vi "Check_with_Jump.vi"(4 "Model       Roll      Pitch       Yaw (deg)":dbl[](array[numeric]) format="%#.2f", 5 "Simulate/Run":T1=enum."Run VI", 6 "Exclude Array":T2[](array[typedef])=[{"Sizes"=[{"Max"=1000.0, "Min"=-1000.0}, {"Max"=1000.0, "Min"=-1000.0}, {"Max"=20.0, "Min"=0.0}], "Name"="Roughness Elements", "Exclude Type"=enum."Allow only vertical moves"}, {"Sizes"=[{"Max"=50.0, "Min"=-50.0}, {"Max"=50.0, "Min"=-50.0}, {"Max"=220.0, "Min"=-0.0}], "Name"="B204", "Exclude Type"=enum."Exclude completely"}] {"Sizes"."Min" format="%#.1f"; "Sizes"."Max" format="%#.1f"}, 7 "Traverse Name":string, 8 "Probe Volume":T3=[{"Max"=10.0, "Min"=-10.0}, {"Max"=10.0, "Min"=-10.0}, {"Max"=200.0, "Min"=0.0}] {"Min" format="%#.1f"; "Max" format="%#.1f"}, 9 "Entire Space":T3=[{"Max"=500.0, "Min"=-500.0}, {"Max"=1000.0, "Min"=-1000.0}, {"Max"=700.0, "Min"=0.0}] {"Min" format="%#.1f"; "Max" format="%#.1f"}, 10 "New Position":dbl[](array[numeric])=[0.0, 100.0, 40.0] format="%.2f", 11 "Current position":dbl[](array[numeric])=[0.0, 200.0, 40.0] format="%.2f") -> (1 "Steps":dbl[][](array[numeric])=[[0.0, 200.0, 40.0]] format="%.2f", 3 "Error Comments":string)   [LabVIEW 2011]
uses:
  Box_size.ctl
  Exclude_cluster.ctl
  Exclusion_type.ctl
  Controls/User_Specific_mode.ctl
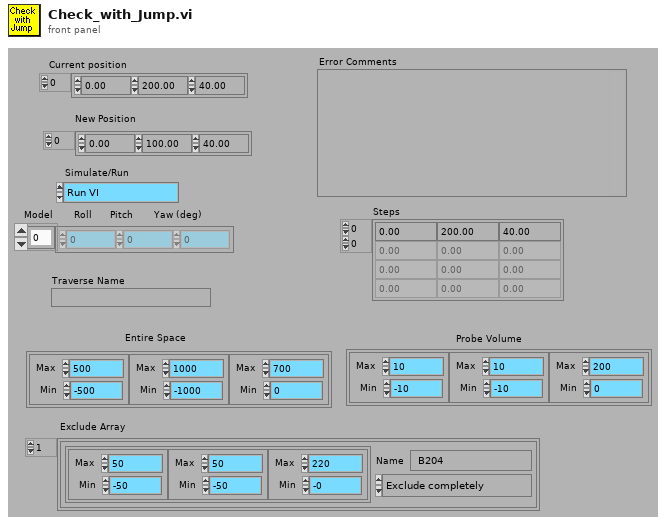
[diagram p1: front panel]
types:
  T1 = typedef "User_Specific_mode.ctl" = enum16{"Check VI only", "Run VI"}
  T2 = typedef "Exclude_cluster.ctl" = cluster{"Sizes":T3, "Name":string, "Exclude Type":T4}
  T3 = typedef "Box_size.ctl" = cluster{"Max":dbl, "Min":dbl}[]
  T4 = typedef "Exclusion_type.ctl" = enum16{"Exclude completely", "Allow only vertical moves"}
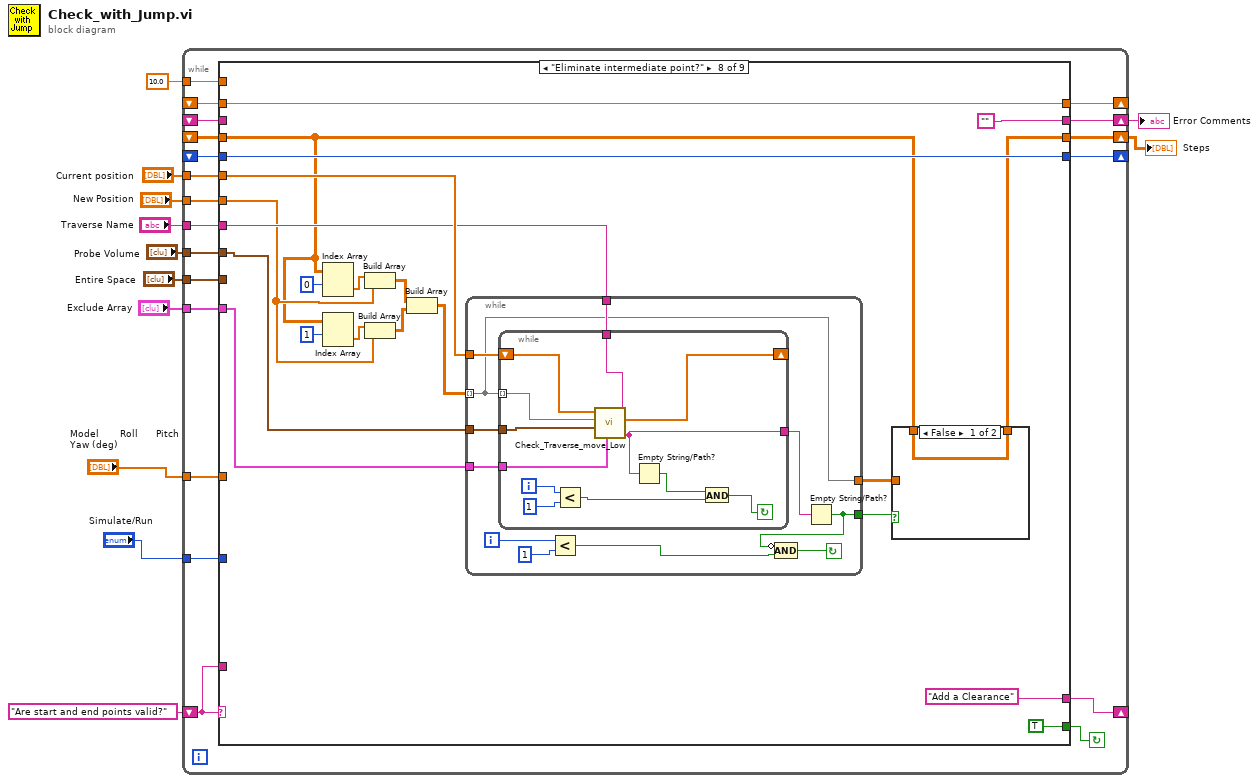
[diagram p0: block diagram]
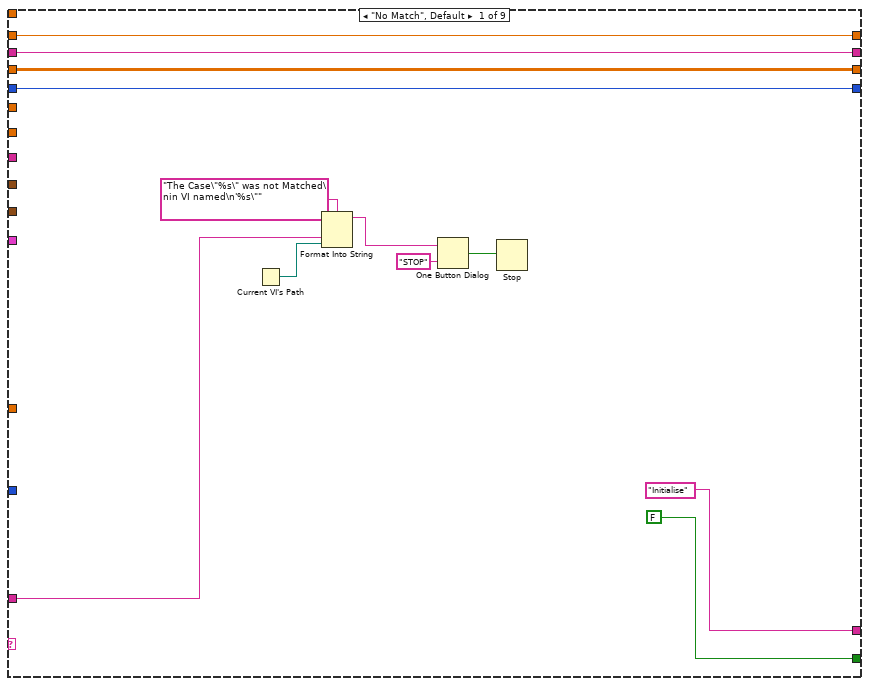
[diagram p2: hidden frame]
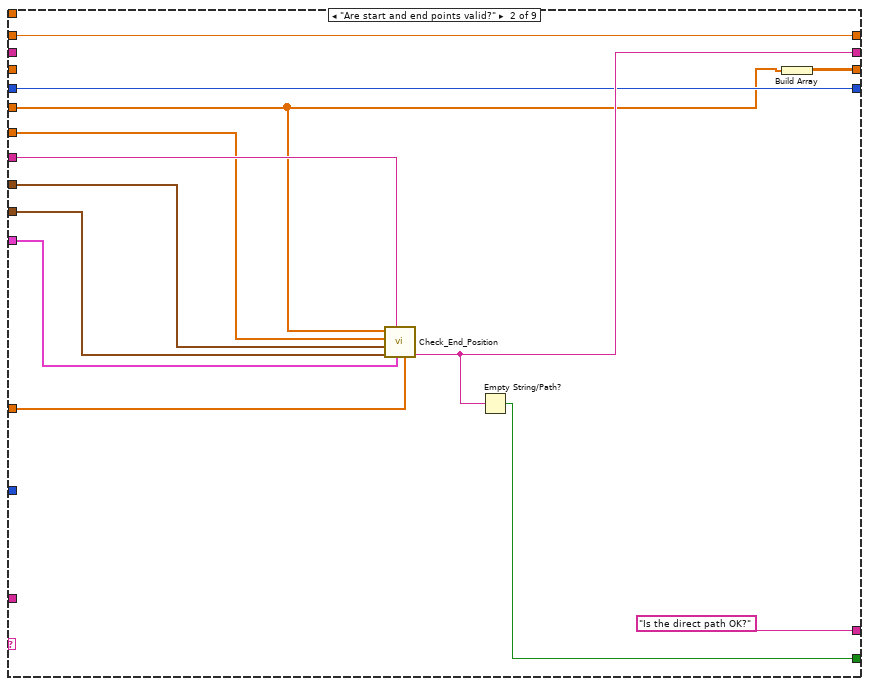
[diagram p3: hidden frame]
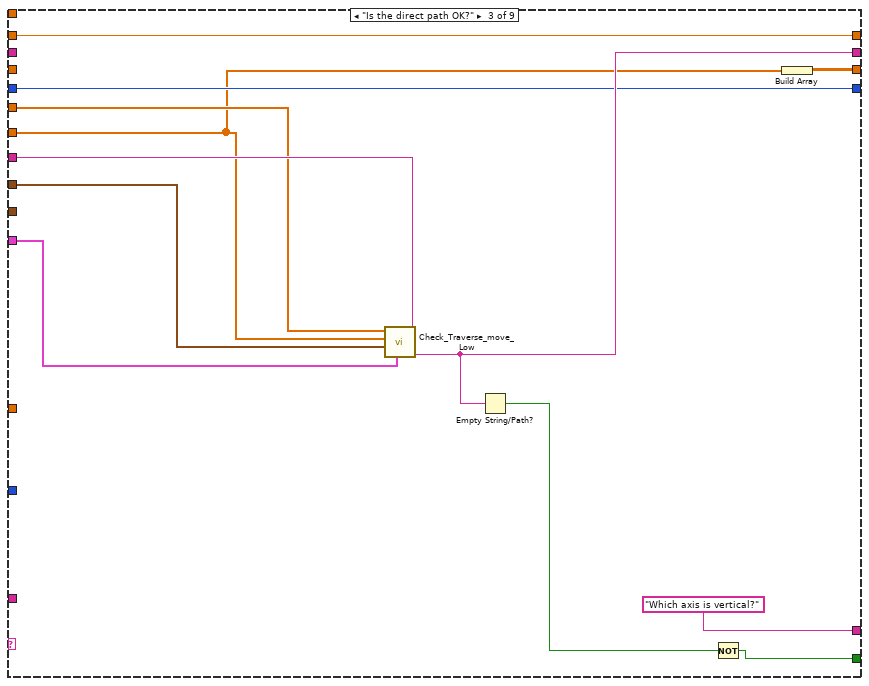
[diagram p4: hidden frame]
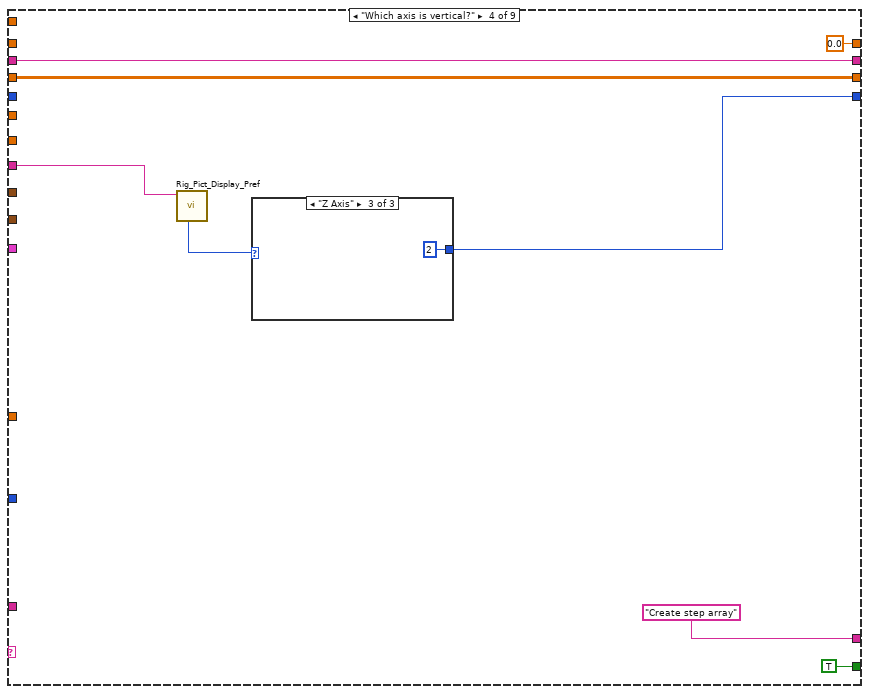
[diagram p5: hidden frame]
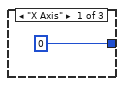
[diagram p6: hidden frame]
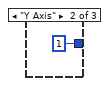
[diagram p7: hidden frame]
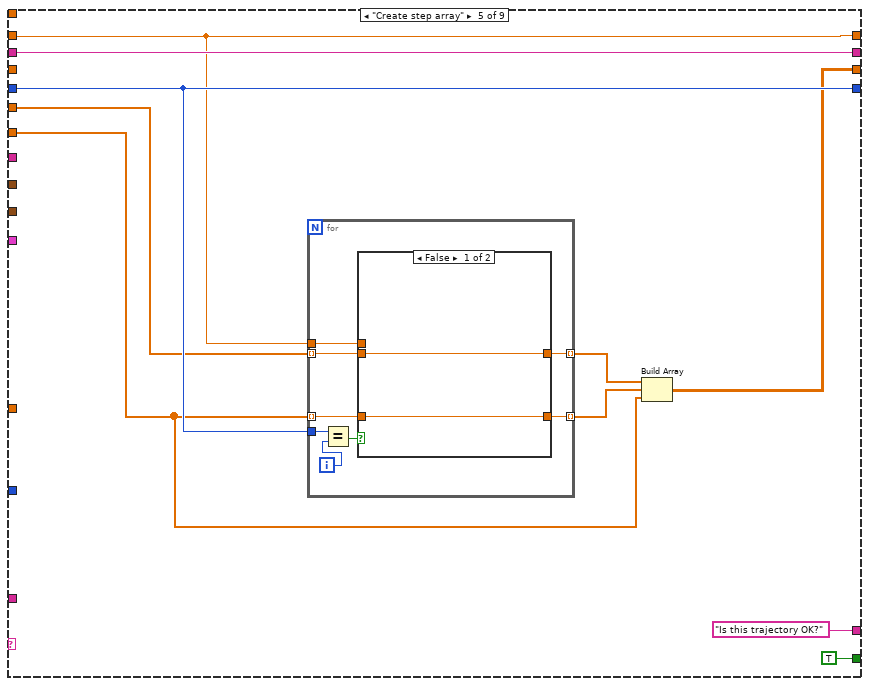
[diagram p8: hidden frame]
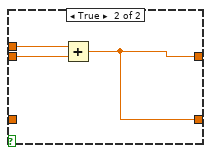
[diagram p9: hidden frame]
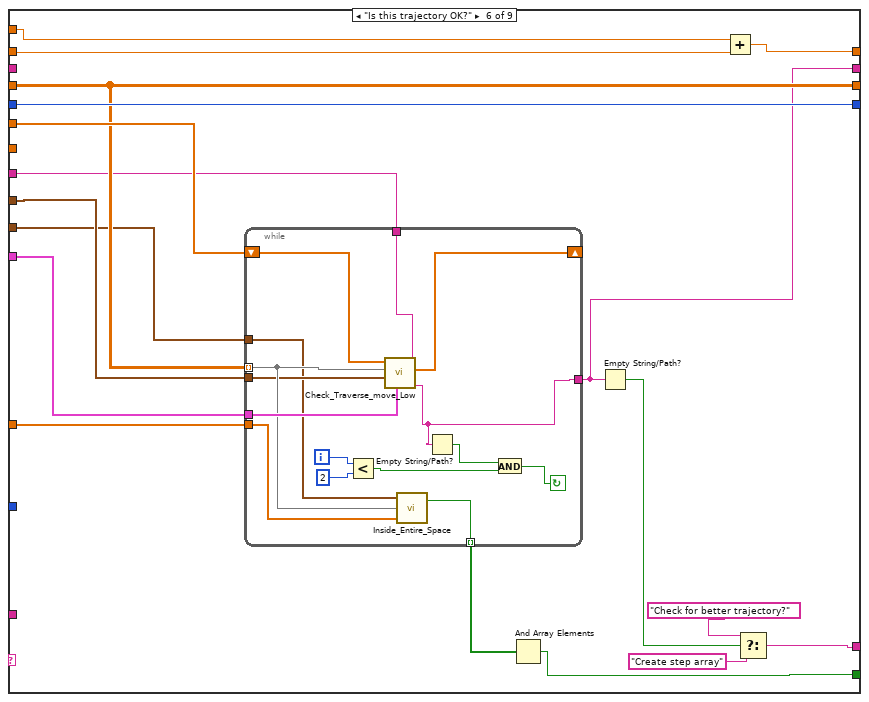
[diagram p10: hidden frame]
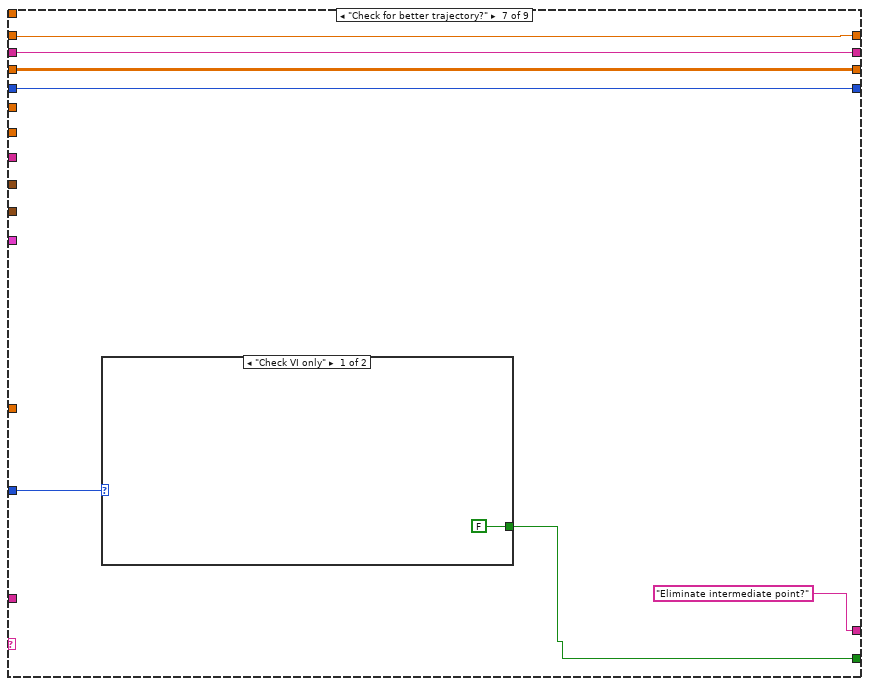
[diagram p11: hidden frame]
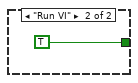
[diagram p12: hidden frame]
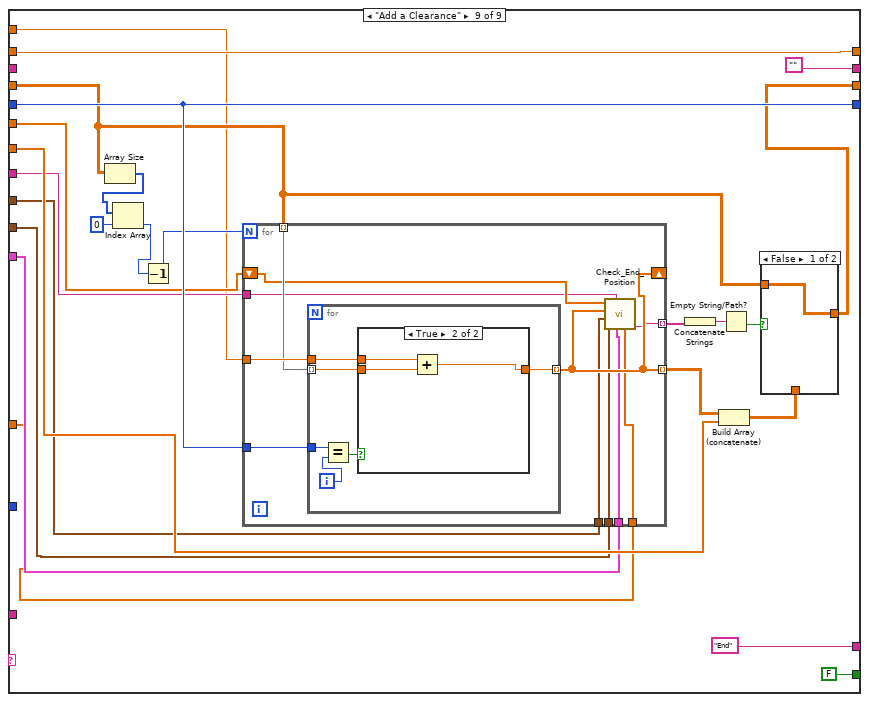
[diagram p14: hidden frame]
diagram:
  n1 = while {
    shift-left: "Are start and end points valid?" -> [w31]
    shift-right: [w32] -> _
    shift-right: [w28] -> w4
    shift-left: _ -> [w29]
    shift-right: [w27] -> w5
    shift-left: _ -> [w26]
    tunnel: "Current position" -> [w25]
    tunnel: "New Position" -> [w24]
    tunnel: "Probe Volume" -> [w23]
    tunnel: "Entire Space" -> [w22]
    tunnel: "Exclude Array" -> [w21]
    tunnel: "Traverse Name" -> [w20]
    shift-right: [w19] -> _
    shift-left: _ -> [w18]
    shift-right: [w17] -> _
    shift-left: _ -> [w16]
    tunnel: 10.0 -> [w15]
    tunnel: "Simulate/Run" -> [w14]
    tunnel: "Model       Roll      Pitch       Yaw (deg)" -> [w13]
    stop <- w30 continue-if-true
    n2 = case shown="\"Eliminate intermediate point?\"" w31 {
      tunnel: [FALSE w50 w61 TRUE TRUE w104 w137 TRUE FALSE] -> w30
      tunnel: ["Initialise" "Is the direct path OK?" "Which axis is vertical?" "Create step array" "Is this trajectory OK?" w114 "Eliminate intermediate point?" "Add a Clearance" "End"] -> w32
      tunnel: w31 -> [w39 _ _ _ _ _ _ _ _]
      tunnel: w29 -> [w36 _ _ w75 w89 _ w143 _ _]
      tunnel: [w36 w52 w65 w75 w89 w111 w143 "" ""] -> w28
      tunnel: [w35 w51 w63 w76 w82 w119 w140 w152 w200] -> w27
      tunnel: w26 -> [w35 _ _ w76 _ w119 w140 w150 w199]
      tunnel: w25 -> [_ w46 w64 _ w86 w120 _ w165 w205]
      tunnel: w24 -> [_ w47 w58 _ w83 _ _ w157 w206]
      tunnel: w23 -> [_ w56 w68 _ _ w118 _ w164 w198]
      tunnel: w22 -> [_ w55 _ _ _ w106 _ _ w197]
      tunnel: w21 -> [_ w54 w67 _ _ w117 _ w163 w196]
      tunnel: w20 -> [_ w53 w66 w74 _ w116 _ w162 w195]
      tunnel: [w34 w49 w60 w72 w87 w121 w142 w166 w213] -> w19
      tunnel: w18 -> [w34 w49 w60 _ w87 w121 w142 w166 w213]
      tunnel: [w33 w48 w59 0.0 w81 w108 w141 w149 w211] -> w17
      tunnel: w16 -> [w33 w48 w59 _ w81 w110 w141 w149 w211]
      tunnel: w15 -> [_ _ _ _ _ w109 _ _ w193]
      tunnel: w14 -> [_ _ _ _ _ _ w139 _ _]
      tunnel: w13 -> [_ w45 _ _ _ w107 _ _ w192]
      frame "No Match", Default {
        n3 = Current VI's Path() -> (path=w38:path)
        n4 = Format Into String(format string="The Case\"%s\" was not Matched\nin VI named\n'%s\"" ("Format String"), w39, w38) -> (resulting string=w42:string)  [unwired: 2 in, 1 out]
        n5 = One Button Dialog(message=w42, button name ("OK")="STOP") -> (true=w40:bool)
        n6 = Stop(stop? (T)=w40) -> ()
      }
      frame "Are start and end points valid?" {
        n7 = call "Check_End_Position.vi"("Model       Roll      Pitch       Yaw (deg)"=w45, "Exclude Array"=w54, "Traverse Name"=w53, "Entire Space"=w55, "Probe Volume"=w56, "New Position"=w47, "Current position"=w46) -> ("Error Comments"=w52:string)  [unwired: 3 out]
        n8 = Empty String/Path?(string/path=w52) -> (empty?=w50:bool)
        n9 = Build Array(w46) -> (w51:dbl[][])
      }
      frame "Is the direct path OK?" {
        n10 = call "Check_Traverse_move_Low.vi"("Traverse Name"=w66, "Exclude Array"=w67, "Probe Volume"=w68, "New Position"=w58, "Current position"=w64) -> ("Error Comments"=w65:string)  [unwired: 1 in, 3 out]
        n11 = Empty String/Path?(string/path=w65) -> (empty?=w62:bool)
        n12 = Not(x=w62) -> (.not. x?=w61:bool)
        n13 = Build Array(w58) -> (w63:dbl[][])
      }
      frame "Which axis is vertical?" {
        n14 = call "Rig_Pict_Display_Pref.vi"("Traverse Name"=w74) -> ("Which Axis is vertical?"=w73:enum16{"X Axis", "Y Axis", "Z Axis"})  [unwired: 7 out]
        n15 = case shown="\"Z Axis\"" w73 {
          tunnel: [0 1 2] -> w72
          frame "X Axis" {
          }
          frame "Y Axis" {
          }
          frame "Z Axis" {
          }
        }
      }
      frame "Create step array" {
        n16 = for {
          tunnel: w81 -> [w98]
          tunnel: w87 -> [w95]
          tunnel: w86 -> [w94] mode=indexing
          tunnel: [w93] -> w85 mode=indexing
          tunnel: w83 -> [w92] mode=indexing
          tunnel: [w91] -> w84 mode=indexing
          i -> [w97]
          n17 = Equal?(x=w95, y=w97) -> (x = y?=w96:bool)
          n18 = case shown="False" w96 {
            tunnel: w98 -> [_ w103]
            tunnel: w94 -> [w100 w102]
            tunnel: [w100 w101] -> w93
            tunnel: w92 -> [w99 _]
            tunnel: [w99 w101] -> w91
            frame False {
            }
            frame True {
              n19 = Add(x=w103, y=w102) -> (x+y=w101:dbl)
            }
          }
        }
        n20 = Build Array(w85, w84, w83) -> (w82:dbl[][])
      }
      frame "Is this trajectory OK?" {
        n21 = while {
          shift-right: [w130] -> _
          shift-left: w120 -> [w131]
          tunnel: w119 -> [w126] mode=indexing
          tunnel: w118 -> [w125]
          tunnel: w117 -> [w128]
          tunnel: w116 -> [w129]
          tunnel: [w127] -> w111
          tunnel: w107 -> [w124]
          tunnel: w106 -> [w122]
          tunnel: [w123] -> w105 mode=indexing
          i -> [w132]
          stop <- w133 continue-if-true
          n22 = Less?(x=w132, y=2 ("x")) -> (x < y?=w134:bool)
          n23 = call "Check_Traverse_move_Low.vi"("Traverse Name"=w129, "Exclude Array"=w128, "Probe Volume"=w125, "New Position"=w126, "Current position"=w131) -> ("Error Comments"=w127:string, "Position At Crash"=w130:dbl[])  [unwired: 1 in, 2 out]
          n24 = call "Inside_Entire_Space.vi"("Model       Roll      Pitch       Yaw (deg)"=w124, "Current Position"=w126, "Envelope"=w122) -> ("Box Inside"=w123:bool)  [unwired: 1 out]
          n25 = Empty String/Path?(string/path=w127) -> (empty?=w135:bool)
          n26 = And(x=w135, y=w134) -> (x .and. y?=w133:bool)
        }
        n27 = And Array Elements(Boolean array=w105) -> (logical AND=w104:bool)
        n28 = Empty String/Path?(string/path=w111) -> (empty?=w115:bool)
        n29 = Add(x=w109, y=w110) -> (x+y=w108:dbl)
        n30 = Select(t="Check for better trajectory?", s=w115, f="Create step array") -> (s? t:f=w114:string)
      }
      frame "Check for better trajectory?" {
        n31 = case shown="\"Check VI only\"" w139 {
          tunnel: [FALSE TRUE] -> w137
          frame "Check VI only" {
          }
          frame "Run VI" {
          }
        }
      }
      frame "Eliminate intermediate point?" {
        n32 = Index Array(array=w150, index (row)=0) -> (element=w159:dbl[])  [unwired: 1 in]
        n33 = Index Array(array=w150, index (row)=1) -> (element=w158:dbl[])  [unwired: 1 in]
        n34 = Build Array(w159, w157) -> (w156:dbl[][])
        n35 = Build Array(w158, w157) -> (w155:dbl[][])
        n36 = Build Array(w156, w155) -> (w154:dbl[][][])
        n37 = while {
          tunnel: w165 -> [w179]
          tunnel: w164 -> [w178]
          tunnel: w163 -> [w177]
          tunnel: w162 -> [w176]
          tunnel: w154 -> [w169] mode=indexing
          tunnel: [w170] -> w153
          tunnel: [w169] -> w151
          i -> [w173]
          stop <- w171 continue-if-true
          n38 = while {
            shift-right: [w187] -> _
            shift-left: w179 -> [w191]
            tunnel: w178 -> [w190]
            tunnel: w177 -> [w189]
            tunnel: w176 -> [w188]
            tunnel: [w181] -> w175
            tunnel: w169 -> [w180] mode=indexing
            i -> [w186]
            stop <- w182 continue-if-true
            n39 = Less?(x=w186, y=1 ("x")) -> (x < y?=w183:bool)
            n40 = call "Check_Traverse_move_Low.vi"("Traverse Name"=w188, "Exclude Array"=w189, "Probe Volume"=w190, "New Position"=w180, "Current position"=w191) -> ("Error Comments"=w181:string, "Position At Crash"=w187:dbl[])  [unwired: 1 in, 2 out]
            n41 = Empty String/Path?(string/path=w181) -> (empty?=w184:bool)
            n42 = And(x=w184, y=w183) -> (x .and. y?=w182:bool)
          }
          n43 = Less?(x=w173, y=1 ("x")) -> (x < y?=w172:bool)
          n44 = Empty String/Path?(string/path=w175) -> (empty?=w170:bool)
          n45 = Compound Arithmetic op=AND(invert w170, w172) -> (w171:bool)
        }
        n46 = case shown="False" w153 {
          tunnel: [w167 w168] -> w152
          tunnel: w151 -> [_ w168]
          tunnel: w150 -> [w167 _]
          frame False {
          }
          frame True {
          }
        }
      }
      frame "Add a Clearance" {
        n47 = Array Size(array=w199) -> (size(s)=w210:i32[])
        n48 = Index Array(array=w210, index=0) -> (element=w208:i32)
        n49 = Decrement(x=w208) -> (x-1=w207:i32)
        n50 = for {
          N: w207 -> [_]
          tunnel: w213 -> [w228]
          tunnel: [w224] -> w212 mode=indexing
          tunnel: w193 -> [w227]
          tunnel: w199 -> [w226] mode=indexing
          shift-right: [w224] -> _
          shift-left: w205 -> [w225]
          tunnel: [w223] -> w204 mode=indexing
          tunnel: w198 -> [w222]
          tunnel: w197 -> [w221]
          tunnel: w196 -> [w220]
          tunnel: w195 -> [w219]
          tunnel: w192 -> [w218]
          n51 = for {
            tunnel: w227 -> [w234]
            tunnel: w228 -> [w231]
            tunnel: w226 -> [w230] mode=indexing
            tunnel: [w229] -> w224 mode=indexing
            i -> [w233]
            n52 = Equal?(x=w231, y=w233) -> (x = y?=w232:bool)
            n53 = case shown="True" w232 {
              tunnel: w234 -> [_ w238]
              tunnel: w230 -> [w235 w237]
              tunnel: [w235 w236] -> w229
              frame False {
              }
              frame True {
                n54 = Add(x=w238, y=w237) -> (x+y=w236:dbl)
              }
            }
          }
          n55 = call "Check_End_Position.vi"("Model       Roll      Pitch       Yaw (deg)"=w218, "Exclude Array"=w220, "Traverse Name"=w219, "Entire Space"=w221, "Probe Volume"=w222, "New Position"=w224, "Current position"=w225) -> ("Error Comments"=w223:string)  [unwired: 3 out]
        }
        n56 = Concatenate Strings(w204) -> (w203:string)
        n57 = Build Array (concatenate)(w212, w206) -> (w201:dbl[][])
        n58 = Empty String/Path?(string/path=w203) -> (empty?=w202:bool)
        n59 = case shown="False" w202 {
          tunnel: w201 -> [_ w217]
          tunnel: [w216 w217] -> w200
          tunnel: w199 -> [w216 _]
          frame False {
          }
          frame True {
          }
        }
      }
    }
  }
  "Error Comments" <- w4
  "Steps" <- w5
